vi "Modualeted Param 14444B UP.vi"(6 "encoder divider":dbl, 8 "Error In":errorcluster, 9 "BIT RATE":dbl, 10 "Bit stream out (NRZ encode)":u8[](array[numeric])) -> (0 "Error Out":errorcluster, 2 "output complex waveform":T1 {"Y" format="%.3f"; "dt" format="%^.2e"; "t0" format="%.4f"})   [LabVIEW 2019]
uses:
  <vilib>/addons/Modulation/Analog/controls/Complex Data Waveform.ctl
  <vilib>/addons/Modulation/Analog/support/mod_Set Error Source.vi
  <vilib>/addons/Modulation/Digital/Support/Common/Validators/mod_Generate Filter Coefficients Validate.vi
  <vilib>/addons/Modulation/Digital/General/subVIs/mod_Generate Filter Coefficients.vi
  <vilib>/addons/Modulation/Digital/General/MT Generate ASK system parameters (M).vi
  <vilib>/addons/Modulation/niDMT.lvlib
  <vilib>/addons/Modulation/niAMT.lvlib
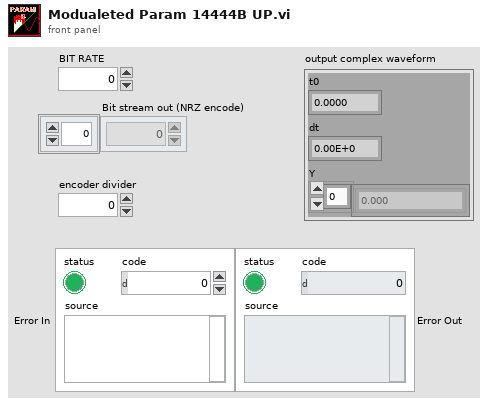
[diagram p1: front panel]
types:
  T1 = typedef "niAMT.lvlib/Complex Data Waveform.ctl" = cluster{"t0":dbl, "dt":dbl, "Y":cdb[]}
  T2 = enum16{"none", "Raised Cosine", "Root Raised Cos", "Gaussian"}
  T3 = enum16{"FSK", "PSK", "QAM", "MSK", "PAM", "ASK", "CPM"}
  T4 = cluster{"samples per symbol (16)":i32, "symbol map":cdb[]}
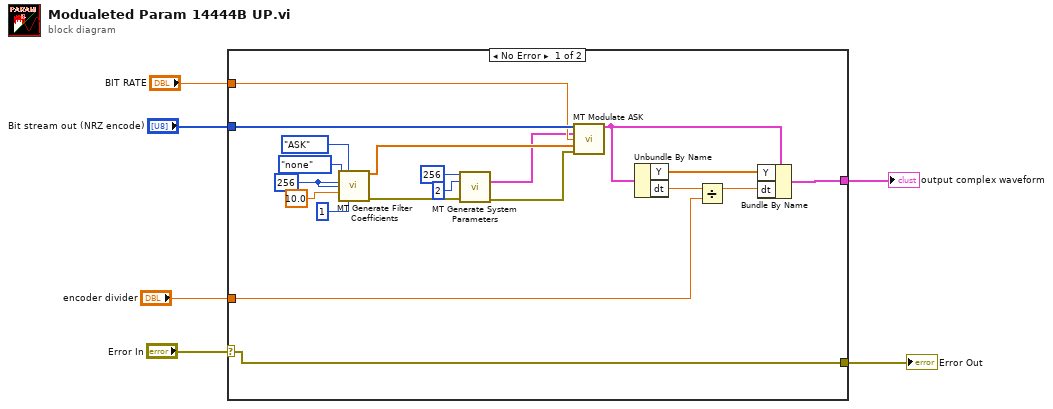
[diagram p0: block diagram]
diagram:
  n1 = case shown="No Error" "Error In" {
    selector: "Error In" -> [w9 w27]
    tunnel: [w26 _] -> w6
    tunnel: "Bit stream out (NRZ encode)" -> [w25 _]
    tunnel: "encoder divider" -> [w23 _]
    tunnel: "BIT RATE" -> [w20 _]
    tunnel: [w9 w27] -> w1
    frame No Error {
      w16 = 256 ("pulse shaping samples per symbol (16)")
      n2 = call <vilib>:"MT Generate Filter Coefficients.vi"("pulse shaping filter (none)"=T2."none", "modulation type"=T3."ASK", "pulse shaping samples per symbol (16)"=w16, "matched samples per symbol (16)"=w16, "filter parameter"=10.0, "filter length (symbols)"=1) -> ("pulse shaping filter coefficients"=w18:dbl[], "error out"=w13:errorcluster)  [unwired: 1 in, 7 out]
      n3 = call-poly <vilib>:"MT Generate System Parameters.vi"("samples per symbol (16)"=256, "M-ASK (2)"=2, "error in (no error)"=w13) -> ("ASK system parameters"=w10:T4, "error out"=w11:errorcluster)  [unwired: 11 out]
      n4 = call <vilib>:"MT Modulate ASK.vi"("input bit stream"=w25, "ASK system parameters"=w10, "symbol rate (Hz)"=w20, "pulse shaping filter coefficients"=w18, "error in (no error)"=w11) -> ("output complex waveform"=w24:T1)  [unwired: 8 in, 2 out]
      n5 = Unbundle By Name(w24) -> ("Y"=w8:cdb[], "dt"=w22:dbl)
      n6 = Divide(x=w22, y=w23) -> (x/y=w21:dbl)
      n7 = Bundle By Name(cluster=w24, "Y"=w8, "dt"=w21) -> (w26:T1)
    }
    frame Error {
    }
  }
  "output complex waveform" <- w6
  "Error Out" <- w1
